vi "Output OFF.vi"(0 "VISA resource name":refnum<visa-resource-name>, 11 "error in (no error)":errorcluster) -> (4 "VISA resource name out":refnum<visa-resource-name>, 15 "error out":errorcluster)   [LabVIEW 2014, in "Associated Power Technologies 8500 Series.lvlib"]
doc: "Stop the instrument during the test process."
uses:
  <instrlib>/Associated Power Technologies 8500 Series/Associated Power Technologies 8500 Series.lvlib
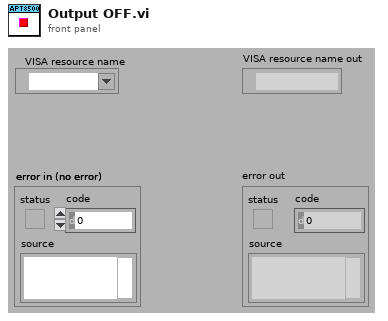
[diagram p1: front panel]
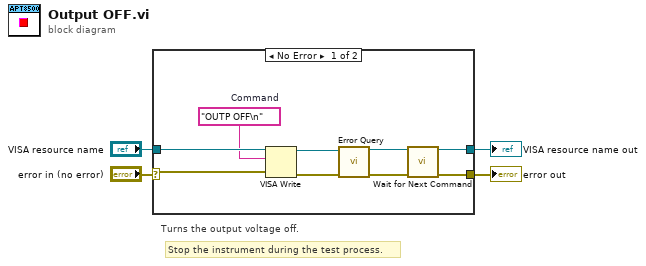
[diagram p0: block diagram]
diagram:
  # "Stop the instrument during the test process."
  # "Turns the output voltage off."
  n1 = case shown="No Error" "error in (no error)" {
    selector: "error in (no error)" -> [w12 w15]
    tunnel: "VISA resource name" -> [w13 w14]
    tunnel: [w9 w14] -> w3
    tunnel: [w10 w15] -> w2
    frame No Error {
      w11 = "OUTP OFF\n"  # Command
      n2 = VISA Write(VISA resource name=w13, write buffer=w11, error in (no error)=w12) -> (VISA resource name out=w6:refnum<visa-resource-name>, error out=w5:errorcluster)  [unwired: 1 out]
      n3 = call <instrlib>:"Error Query.vi"("VISA resource name"=w6, "error in (no error)"=w5) -> ("VISA resource name out"=w8:refnum<visa-resource-name>, "error out"=w7:errorcluster)  [unwired: 10 in, 2 out]
      n4 = call <instrlib>:"Wait for Next Command.vi"("VISA resource name"=w8, "error in (no error)"=w7) -> ("VISA resource name out"=w9:refnum<visa-resource-name>, "error out"=w10:errorcluster)  [unwired: 12 in]
    }
    frame Error {
    }
  }
  "error out" <- w2
  "VISA resource name out" <- w3
